vi "MAIN - Template Application.vi"() -> ()   [LabVIEW 2015, in "TLB` Template.lvlib"]
doc: "TLB Prime - Application Template 1.3.0.24\nNorm Kirchner, NI Systems Engineering - NI\nCopyright (c) 2014, NI"
uses:
  TLB` Template.lvlib
  State Declaration.ctl
  System Trigger.ctl
  System Trigger Element.ctl
  <vilib>/Utility/error.llb/DialogTypeEnum.ctl
  Read Termination Message.vi
  Update Message Routing Info.vi
  Create Multiple Messages.vi
  Create Single Message.vi
  TypeDef - SHIFTER.ctl
  Globals.vi
  Send Message.vi
  TLB`_Dependencies.lvlib
  AMC.lvlib
panel:
  out "error out":errorcluster
  # "TLB` Template"
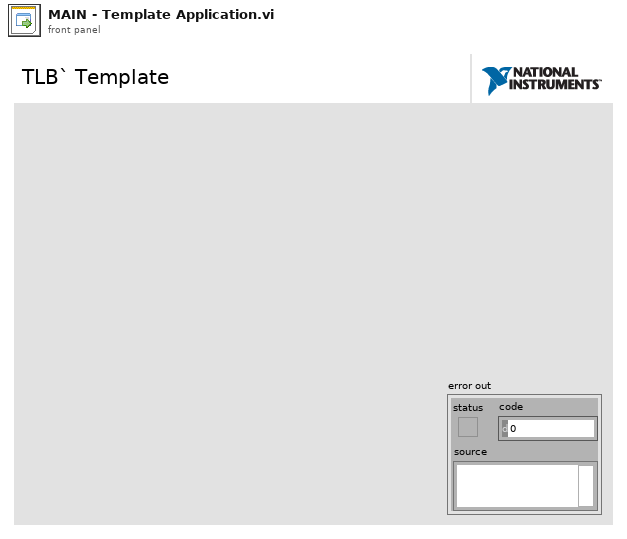
[diagram p1: front panel]
types:
  T1 = typedef "TLB` Template.lvlib/System Trigger.ctl" = enum16{"<None>", "Cache User Parameters", "Close Application"}
  T2 = typedef "TLB` Template.lvlib/State Declaration.ctl" = enum16{"<Startup>", "Idle", "<Shutdown>"}
  T3 = enum16{"Clear SR", "Set Display", "Set Shifter", "Initialize Events", "Init Q"}
  T4 = typedef "TLB` Template.lvlib/TypeDef - SHIFTER.ctl" = cluster{"State":T2, "User Data":cluster{"Active Item Tag":string}, "Display Data":cluster{"Active Item Tag":string}, "User Parameter Controls":refnum<vi>[], "Framework Data":cluster{"Exit Event":T5, "Terminate Error":errorcluster}, "Private Data":cluster{"Active Item Tag":string}}
  T5 = typedef "TLB` Template.lvlib/TLB`_Dependencies.lvlib/Exit Event Ref.ctl" = refnum<user-event>
  T6 = typedef "TLB` Template.lvlib/System Trigger Element.ctl" = cluster{"System Triggers":T1, "Trigger Data":variant}
  T7 = typedef "TLB` Template.lvlib/AMC.lvlib/Message Queue.ctl" = refnum<queue>
  T8 = typedef "DialogTypeEnum.ctl" = enum16{"no dialog", "OK message", "continue or stop message", "auto error handling dialog", "OK message + warnings", "continue/stop + warnings"}
  T9 = enum32{"Invalid", "Standard", "Closed", "Hidden", "Minimized", "Maximized"}
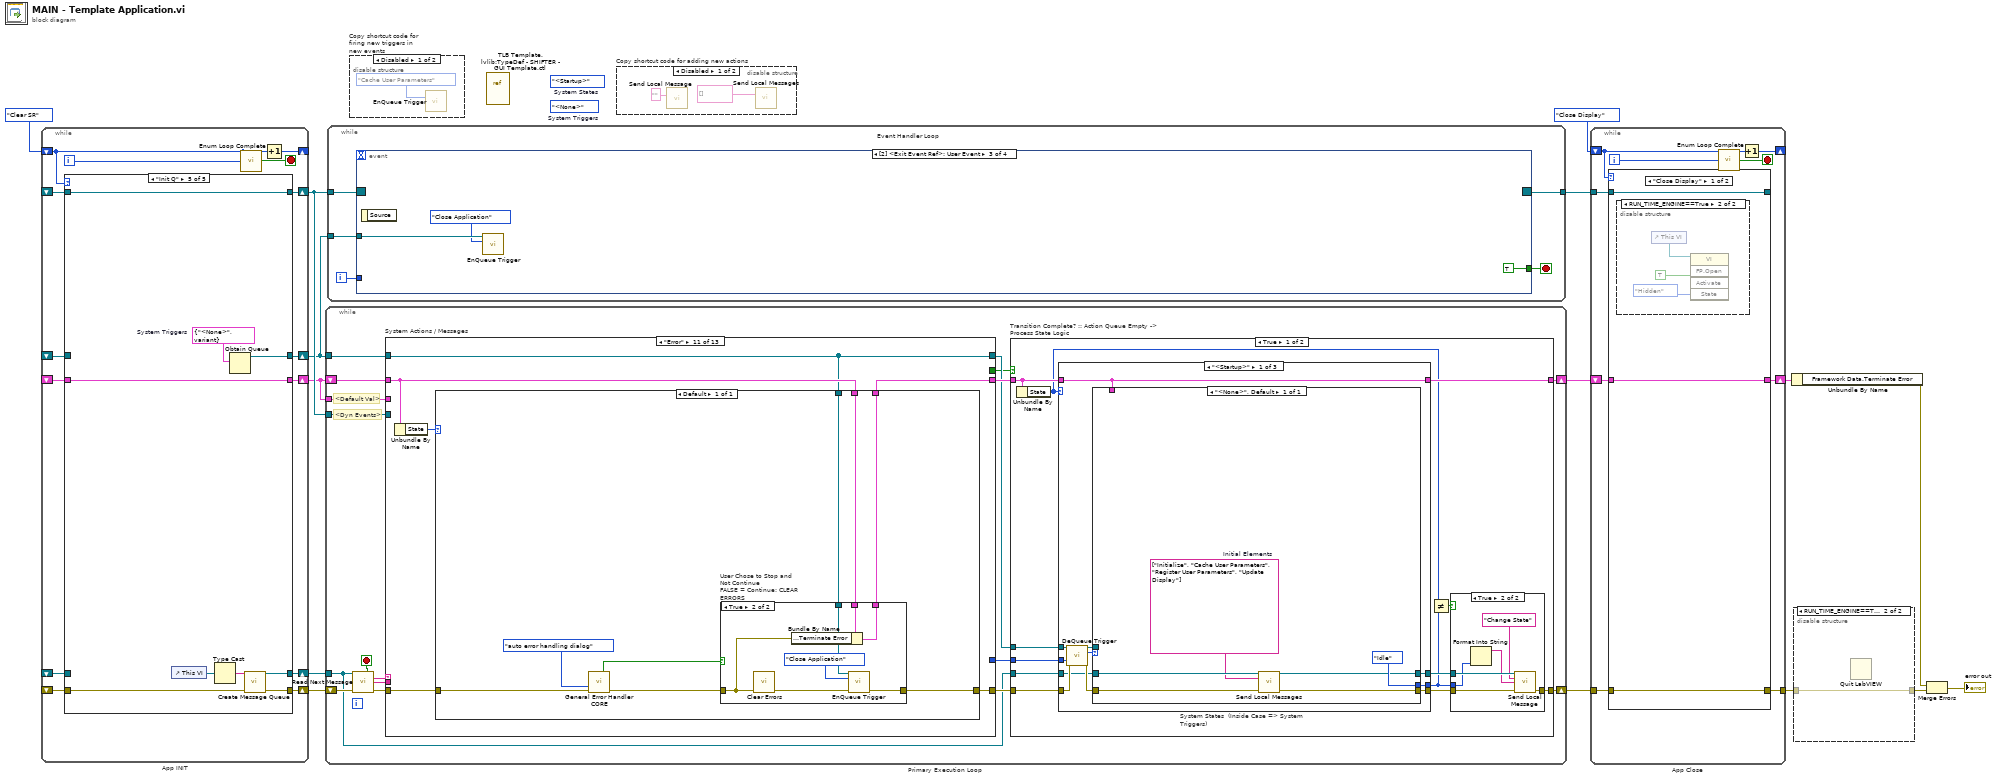
[diagram p0: block diagram]
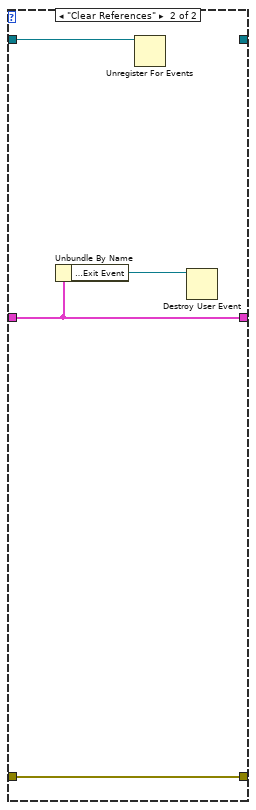
[diagram p6: hidden frame]
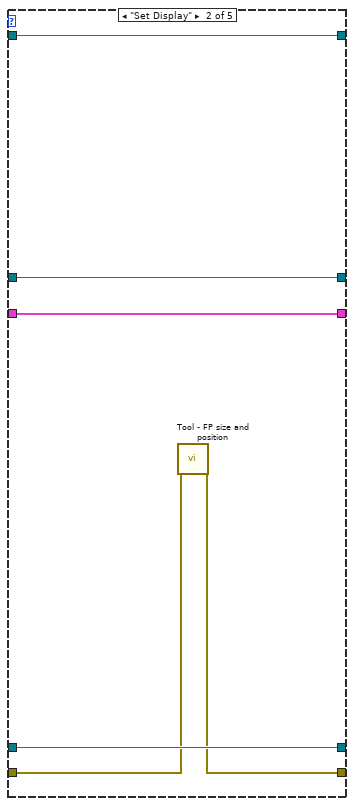
[diagram p8: hidden frame]
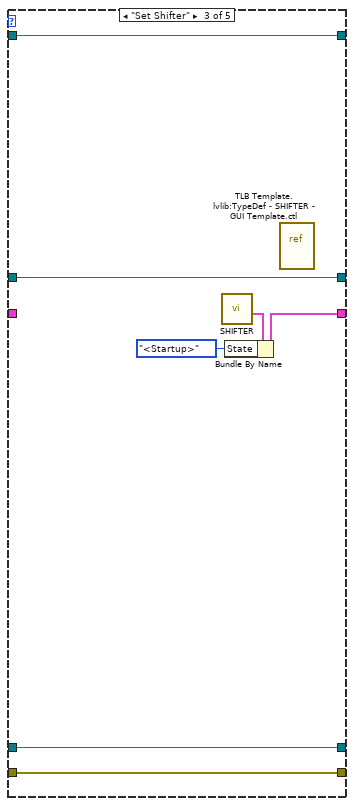
[diagram p9: hidden frame]
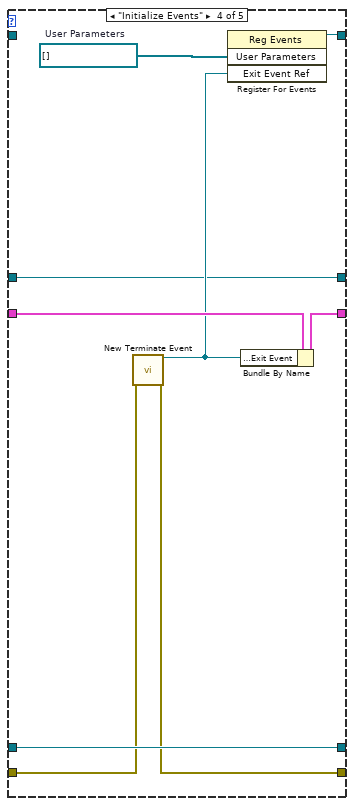
[diagram p10: hidden frame]
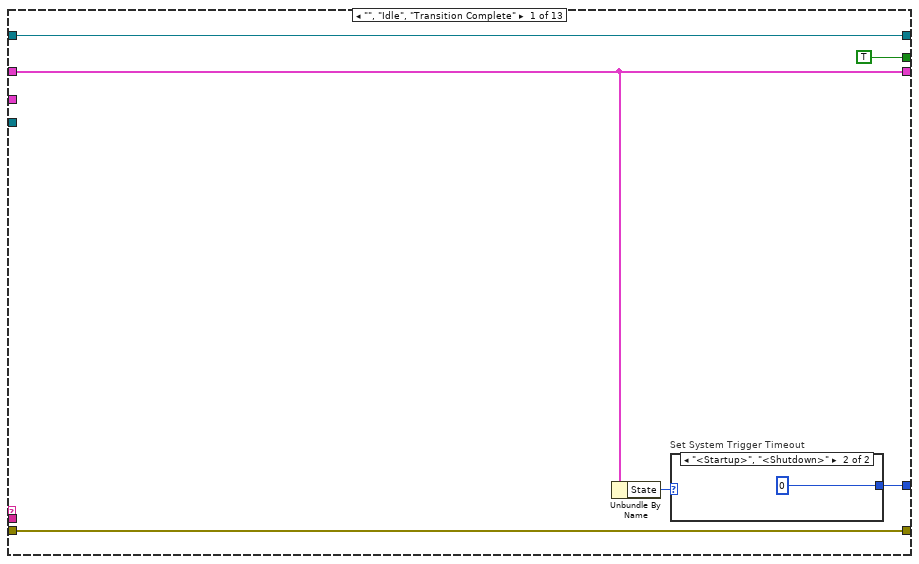
[diagram p11: hidden frame]
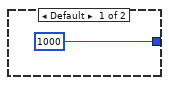
[diagram p12: hidden frame]
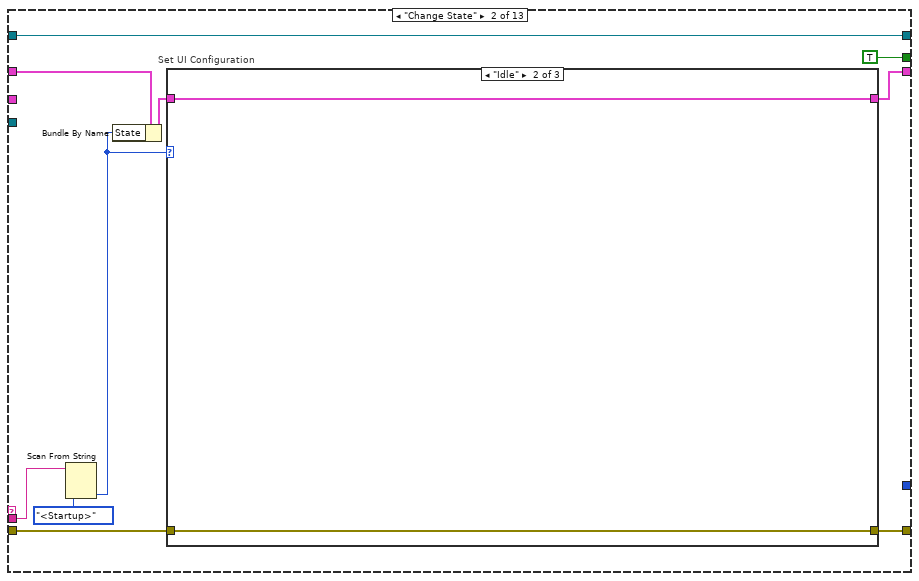
[diagram p13: hidden frame]
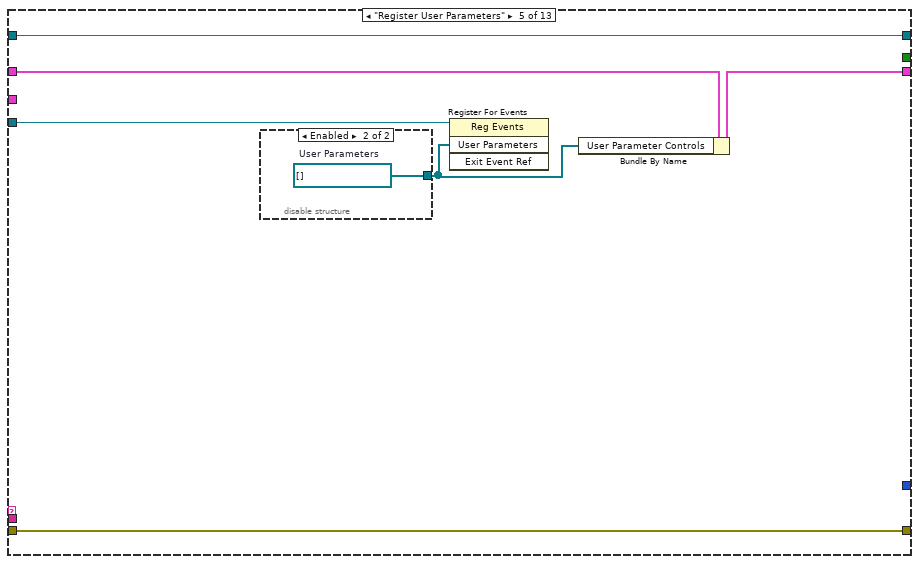
[diagram p18: hidden frame]
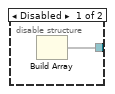
[diagram p19: hidden frame]
diagram:
  (unwired) System_Trigger."<None>"  # System Triggers
  (unwired) State_Declaration."<Startup>"  # System States
  n1 = while "App INIT" {
    shift-right: [w23] -> _
    shift-left: T3."Clear SR" -> [w18]
    shift-right: [w29] -> w9
    shift-left: _ -> [w22]
    shift-right: [w26] -> w8
    shift-left: _ -> [w21]
    shift-right: [w28] -> w11
    shift-left: _ -> [w20]
    shift-right: [w27] -> w1
    shift-left: _ -> [w19]
    shift-right: [w17] -> w2
    shift-left: _ -> [w16]
    i -> [w24]
    stop <- w25 stop-if-true
    n2 = case shown="\"Init Q\"" w18 {
      tunnel: [_ w33 w42 w51 w56] -> w29
      tunnel: [_ w31 w41 w44 w55] -> w26
      tunnel: [_ w35 w36 w48 w54] -> w27
      tunnel: [_ w34 w40 w47 w60] -> w28
      tunnel: w22 -> [_ w33 w42 w51 _]
      tunnel: w21 -> [_ w32 w41 w45 w59]
      tunnel: w20 -> [_ w34 w40 _ w60]
      tunnel: w19 -> [_ w35 _ w49 w54]
      tunnel: [_ w30 w39 w43 w58] -> w17
      tunnel: w16 -> [_ w30 w39 w43 _]
      frame "Clear SR" {
      }
      frame "Set Display" {
        n3 = call "Tool - FP size and position.vi"("error in (no error)"=w32) -> ("error out"=w31:errorcluster)  [unwired: 7 in, 11 out]
      }
      frame "Set Shifter" {
        n4 = call "SHIFTER.vi"() -> ("SHIFTER DATA"=w37:T4)  [unwired: 15 in]
        n5 = Bundle By Name(cluster=w37, "State"=State_Declaration."<Startup>") -> (w36:T4)
        n6 = vi-ref "TLB Template.lvlib:TypeDef - SHIFTER - GUI Template.ctl"() -> ()  [unwired: 1 out]
      }
      frame "Initialize Events" {
        w50 = refnum<vi>[] []  # User Parameters
        n7 = call "New Terminate Event.vi"("error in (no error)"=w45) -> ("Exit Event Ref"=w46:T5, "error out"=w44:errorcluster)  [unwired: 13 in]
        n8 = register-events(w50, w46) -> (reference out=w47:refnum<event-registration>)  [unwired: 2 in, 1 out]
        n9 = Bundle By Name(cluster=w49, "Framework Data.Exit Event"=w46) -> (w48:T4)
      }
      frame "Init Q" {
        w57 = T6 {"System Triggers"=enum."<None>", "Trigger Data"=variant}  # System Triggers
        n10 = control-ref of="This VI"() -> (w53:refnum<vi>)
        n11 = Type Cast(x=w53) -> (*(type *) &x=w52:string)  [unwired: 1 in]
        n12 = Obtain Queue(element data type=w57) -> (queue out=w58:refnum<queue>)  [unwired: 4 in, 2 out]
        n13 = call "Create Message Queue.vi"("message queue name"=w52, "error in"=w59) -> ("message queue out"=w56:T7, "error out"=w55:errorcluster)  [unwired: 12 in]
      }
    }
    n14 = call "Enum Loop Complete.vi"("Current State Enum"=w18, "Itteration"=w24) -> ("Loop Complete?"=w25:bool)  [unwired: 13 out]
    n15 = Increment(x=w18) -> (x+1=w23:T3)
  }
  n16 = while "Primary Execution Loop" {
    shift-right: [w67] -> w15
    shift-left: w8 -> [w74]
    shift-right: [w70] -> w14
    shift-left: w1 -> [w77]
    tunnel: w1 -> [w76]
    tunnel: w9 -> [w65]
    tunnel: w11 -> [w75]
    tunnel: w2 -> [w66]
    stop <- w72 stop-if-true
    # "<Dyn Events>"
    # "<Default Val>"
    n17 = call "Read Next Message.vi"("message queue in"=w65, "error in"=w74) -> ("exit process?"=w72:bool, "message name"=w71:string, "message value"=w62:string, "error out"=w73:errorcluster)  [unwired: 6 in, 4 out]
    n18 = case "System Actions / Messages" shown="\"Error\"" w71 {
      selector: w71 -> [_ _ _ _ _ _ _ _ _ _ _ _ w166]
      tunnel: [w83 w90 w104 w105 w113 w118 w121 w126 w129 w132 w137 w160 w170] -> w68
      tunnel: w73 -> [w83 w89 w104 w105 w113 w118 w121 w126 w129 w132 w138 w159 w171]
      tunnel: w77 -> [w78 w86 w103 w107 w112 w117 w123 w125 w128 w131 w135 w163 w172]
      tunnel: w76 -> [_ _ _ _ _ _ _ _ _ _ _ _ _]
      tunnel: [w78 w88 w103 w107 w111 w117 w122 w125 w128 w131 w136 w163 w172] -> w69
      tunnel: [w79 _ _ _ _ _ _ _ _ _ _ _ _] -> w61
      tunnel: w75 -> [_ _ _ _ w110 _ _ _ _ _ _ _ _]
      tunnel: [w81 w94 w102 w106 w109 w116 w120 w124 w127 w130 w133 w157 w164] -> w64
      tunnel: w66 -> [w81 w94 w102 w106 w109 w116 w120 w124 w127 w130 w133 w157 w164]
      tunnel: [TRUE TRUE _ _ _ _ _ _ _ _ _ _ _] -> w63
      tunnel: w62 -> [_ w93 _ _ _ _ _ _ _ _ _ _ _]
      frame "", "Idle", "Transition Complete" {
        n19 = Unbundle By Name(w78) -> ("State"=w80:T2)
        n20 = case "Set System Trigger Timeout" shown="\"<Startup>\", \"<Shutdown>\"" w80 {
          tunnel: [1000 0] -> w79
          frame Default {
          }
          frame "<Startup>", "<Shutdown>" {
          }
        }
      }
      frame "Change State" {
        n21 = Scan From String(input string=w93, default 1=State_Declaration."<Startup>" ("State")) -> (output 1=w91:T2)  [unwired: 3 in, 3 out]
        n22 = Bundle By Name(cluster=w86, "State"=w91) -> (w87:T4)
        n23 = case "Set UI Configuration" shown="\"Idle\"" w91 {
          tunnel: [w96 w99 w101] -> w90
          tunnel: w89 -> [w96 w99 w101]
          tunnel: [w97 w98 w100] -> w88
          tunnel: w87 -> [w97 w98 w100]
          frame "<Startup>" {
          }
          frame "Idle" {
          }
          frame "<Shutdown>" {
          }
        }
      }
      frame "/*********Initialize********/" {
      }
      frame "Initialize" {
      }
      frame "Register User Parameters" {
        n24 = disable-structure shown="Enabled" {
          disable-tunnel: [w114 w115] -> w108
          frame Disabled {
            n25 = Build Array() -> (w114:void[])  [unwired: 3 in]
          }
          frame Enabled {
            w115 = refnum<vi>[] []  # User Parameters
          }
        }
        n26 = register-events(reference=w110, w108) -> ()  [unwired: 2 in, 2 out]
        n27 = Bundle By Name(cluster=w112, "User Parameter Controls"=w108) -> (w111:T4)
      }
      frame "/*********Display Updates********/" {
      }
      frame "Cache User Parameters" {
        n28 = Bundle By Name(cluster=w123, "User Data.Active Item Tag"="") -> (w122:T4)
      }
      frame "Update Display" {
      }
      frame "/*********Primary Execution********/" {
      }
      frame "/*********Shutdown********/" {
      }
      frame "Error" {
        n29 = Unbundle By Name(w135) -> ("State"=w134:T2)
        n30 = case shown="Default" w134 {
          tunnel: w138 -> [w146]
          tunnel: [w145] -> w137
          tunnel: w135 -> [w142]
          tunnel: [w141] -> w136
          tunnel: w133 -> [w139]
          frame Default {
            n31 = call <vilib>:"General Error Handler CORE.vi"("type of dialog (OK msg:1)"=DialogTypeEnum."auto error handling dialog", "error in (no error)"=w146) -> ("stop event propagated"=w144:bool, "error out"=w140:errorcluster)  [unwired: 12 out]
            n32 = case "User Chose to Stop and Not Continue\nFALSE = Continue: CLEAR ERRORS" shown="True" w144 {
              tunnel: [w147 w152] -> w145
              tunnel: w140 -> [w148 w154]
              tunnel: w142 -> [w149 w156]
              tunnel: [w149 w155] -> w141
              tunnel: w139 -> [_ w153]
              frame False {
                n33 = call <vilib>:"Clear Errors.vi"("error in (no error)"=w148) -> ("error out"=w147:errorcluster)  [unwired: 1 in, 5 out]
              }
              frame True {
                n34 = call <vilib>:"Clear Errors.vi"("error in (no error)"=w154) -> ("error out"=w151:errorcluster)  [unwired: 1 in, 5 out]
                n35 = Bundle By Name(cluster=w156, "Framework Data.Terminate Error"=w154) -> (w155:T4)
                n36 = call "EnQueue Trigger.vi"("Queue in"=w153, "System Triggers"=System_Trigger."Close Application", "error in (no error)"=w151) -> ("error out"=w152:errorcluster)  [unwired: 11 in, 1 out]
              }
            }
          }
        }
      }
      frame "Exit" {
        w158 = refnum<class> refnum  # event data
        # "Don't wire 'Error In'\nMust Execute Regardless"
        n37 = Unbundle By Name(w163) -> ("Framework Data.Exit Event"=w162:T5)  [unwired: 1 out]
        n38 = Generate User Event(user event=w162, event data cluster=w158) -> (error out=w161:errorcluster)  [unwired: 2 in, 1 out]
        n39 = Merge Errors(w161, w159) -> (w160:errorcluster)
      }
      frame Default {
        w168 = 1 items=["No error", "Argument error", "Memory is full", "Out of zone", "End of file", "File already open", "Generic file I/O error", "File not found", "File permission error", "Disk is full", "Duplicate path", "Too many files open", "System feature not enabled", "Resource file not found", "Cannot add resource", "Resource not found", "Image not found", "Image memory error", "Pen does not exist", "Config type invalid", "Config token not found", "Config parse error", "Config memory error", "Bad external code format", "Bad external code offset", "External code not present", "Null window", "Destroy window error", "Null menu", "Print aborted", "Bad print record", "Print driver error", "Windows error during printing", "Memory error during printing", "Print dialog error", "Generic print error", "Invalid device refnum", "Device not found", "Device parameter error", "Device unit error", "Cannot open device", "Device call aborted", "Generic error", "Cancelled by user", "Object ID too low", "Object ID too high", "Object not in heap", "Unknown heap", "Unknown object (invalid DefProc)", "Unknown object (DefProc not in table)", "Message out of range", "Invalid (null) method", "Unknown message", "Manager call not supported", "Bad address", "Network operation in progress", "Network operation timed out", "Connection is busy", "Network attribute not supported", "Network error", "Address in use", "System out of memory", "Connection aborted", "Connection refused", "Not connected", "Already connected", "Connection closed", "Initialization error (interapplication manager)", "Bad occurrence", "Wait on unbound occurrence handler", "Occurrence queue overflow", "Datalog type conflict", "Unused", "Unrecognized type (interapplication manager)", "Memory corrupt", "Failed to make temporary DLL", "Old CIN version", "Drag socket not found", "Failed to load drop-object", "Failed to register OLE object", "Failed to release OLE object", "Format specifier type mismatch", "Unknown format specifier", "Too few format specifiers", "Too many format specifiers", "Scan failed", "Newer CIN version", "Error converting to variant", "Runtime menu error", "Password tampered", "Variant attribute not found", "Incompatible variant data type", "Event data is not available", "Event Store is not present", "Occurrence is not found", "Event Queue is not created", "Event info is not available", "Refnum passed is NULL", "Error retrieving Class GUID", "Error retrieving CoClass GUID", "Error retrieving TypeLib GUID.", "Bad built application magic bytes.", "Specific driver is different from the specific driver associated with the Logical Name.", "There is no session opened to the class driver.", "Max Error", "MAX - Error with config objects", "MAX - Error loading configuration", "MAX - Group not supported"]
        w169 = TRUE  # status
        n40 = Format Into String(format string="DEVELOPER ERROR:\nImproper Action Requested\n================\nAction {%s} does not exist within this architecture\n\nCheck for spelling and case errors" ("source"), w166) -> (resulting string=w167:string)  [unwired: 2 in, 1 out]
        n41 = Bundle By Name(cluster=w171, "status"=w169, "code"=w168, "source"=w167) -> (w170:errorcluster)
      }
    }
    n42 = case "Transition Complete? :: Action Queue Empty -> Process State Logic" shown="True" w63 {
      tunnel: [w184 w254] -> w70
      tunnel: w69 -> [w174 w254]
      tunnel: w68 -> [w183 w253]
      tunnel: w65 -> [w182 _]
      tunnel: [w178 w253] -> w67
      tunnel: w64 -> [w181 _]
      tunnel: w61 -> [w175 _]
      frame True {
        n43 = Unbundle By Name(w174) -> ("State"=w173:T2)
        n44 = case "System States  (Inside Case => System Triggers)" shown="\"<Startup>\"" w173 {
          selector: w173 -> [_ w213 _]
          tunnel: [w200 w219 w244] -> w184
          tunnel: w174 -> [w200 w219 w244]
          tunnel: w183 -> [w194 w211 w238]
          tunnel: w182 -> [w192 w215 w236]
          tunnel: [w199 w218 w243] -> w179
          tunnel: w181 -> [w202 w220 w246]
          tunnel: [w198 w217 w242] -> w180
          tunnel: [w197 w216 w241] -> w177
          tunnel: w175 -> [w196 w209 w240]
          frame "<Startup>" {
            n45 = call "DeQueue Trigger.vi"("Queue in"=w202, "Timeout (0)"=w196, "error in (no error)"=w194) -> ("Queue out"=w195:refnum<queue>, "System Triggers"=w201:T1, "error out"=w193:errorcluster)  [unwired: 9 in, 1 out]
            n46 = case shown="\"<None>\", Default" w201 {
              tunnel: w200 -> [_]
              tunnel: [w206] -> w199
              tunnel: w193 -> [w207]
              tunnel: w192 -> [w205]
              tunnel: [w204] -> w198
              tunnel: [State_Declaration."Idle" ("State")] -> w197
              tunnel: w195 -> [_]
              frame "<None>", Default {
                w203 = string[] ["Initialize", "Cache User Parameters", "Register User Parameters", "Update Display"]  # Initial Elements
                n47 = call "Send Local Messages.vi"("message queue in"=w205, "message names"=w203, "error in"=w207) -> ("message queue out"=w204:T7, "error out"=w206:errorcluster)  [unwired: 10 in, 1 out]
              }
            }
          }
          frame "Idle" {
            n48 = call "DeQueue Trigger.vi"("Queue in"=w220, "Timeout (0)"=w209, "error in (no error)"=w211) -> ("Queue out"=w214:refnum<queue>, "System Triggers"=w212:T1, "error out"=w210:errorcluster)  [unwired: 9 in, 1 out]
            n49 = case shown="\"Cache User Parameters\"" w212 {
              tunnel: w219 -> [_ _ _ _]
              tunnel: [w221 w225 w229 w234] -> w218
              tunnel: w210 -> [w221 w225 w232 w234]
              tunnel: w215 -> [w222 w226 w231 w235]
              tunnel: [w222 w226 w230 w235] -> w217
              tunnel: [State_Declaration."Idle" ("State") State_Declaration."<Shutdown>" ("State") w227 State_Declaration."Idle" ("State")] -> w216
              tunnel: w214 -> [_ _ _ _]
              tunnel: w213 -> [_ _ w227 _]
              frame "<None>" {
              }
              frame "Close Application" {
              }
              frame "Cache User Parameters" {
                n50 = call "Send Local Message.vi"("message queue in"=w231, "message name"="Cache User Parameters" ("Message Name"), "error in"=w232) -> ("message queue out"=w230:T7, "error out"=w229:errorcluster)  [unwired: 10 in, 1 out]
              }
              frame Default {
              }
            }
          }
          frame "<Shutdown>" {
            n51 = call "DeQueue Trigger.vi"("Queue in"=w246, "Timeout (0)"=w240, "error in (no error)"=w238) -> ("Queue out"=w239:refnum<queue>, "System Triggers"=w245:T1, "error out"=w237:errorcluster)  [unwired: 9 in, 1 out]
            n52 = case shown="\"<None>\", Default" w245 {
              tunnel: w244 -> [_]
              tunnel: [w247] -> w243
              tunnel: w237 -> [w249]
              tunnel: w236 -> [w250]
              tunnel: [w248] -> w242
              tunnel: [State_Declaration."<Shutdown>" ("State")] -> w241
              tunnel: w239 -> [_]
              frame "<None>", Default {
                n53 = call "Send Local Messages.vi"("message queue in"=w250, "message names"=string[] ["Exit"], "error in"=w249) -> ("message queue out"=w248:T7, "error out"=w247:errorcluster)  [unwired: 10 in, 1 out]
              }
            }
          }
        }
        n54 = Not Equal?(x=w173, y=w177) -> (x != y?=w176:bool)
        n55 = case shown="True" w176 {
          tunnel: w180 -> [_ w191]
          tunnel: w179 -> [w185 w190]
          tunnel: [w185 w189] -> w178
          tunnel: w177 -> [_ w187]
          frame False {
          }
          frame True {
            n56 = Format Into String(w187) -> (resulting string=w186:string)  [unwired: 3 in, 1 out]
            n57 = call "Send Local Message.vi"("message queue in"=w191, "message name"="Change State" ("Message Name"), "message value"=w186, "error in"=w190) -> ("error out"=w189:errorcluster)  [unwired: 9 in, 2 out]
          }
        }
      }
      frame False {
      }
    }
  }
  n58 = while "Event Handler Loop" {
    tunnel: w11 -> [w258]
    tunnel: [w257] -> w13
    tunnel: w2 -> [w255]
    i -> [w256]
    stop <- w259 stop-if-true
    n59 = event shown="[2] <Exit Event Ref>: User Event" {
      selector: w258 -> [_ _ _ _]
      dyn-events: [_ _ _ _] -> w257
      timeout: _ -> [_ _ _ _]
      tunnel: [_ _ TRUE ("NewVal") _] -> w259
      tunnel: w256 -> [_ _ _ _]
      tunnel: w255 -> [w261 _ w273 w277]
      event Panel Close? {
        w262 = TRUE  # Discard?
        n60 = event-data() -> ()  [unwired: 2 out]
        n61 = call "EnQueue Trigger.vi"("Queue in"=w261, "System Triggers"=System_Trigger."Close Application") -> ()  [unwired: 12 in, 2 out]
        n62 = event-data("Discard?"=w262) -> ()  [unwired: 1 in, 1 out]
      }
      event Mouse Down {
        n63 = event-data() -> ("Button"=w267:u16, "Mods"=w268:cluster{"Double Click":bool, "Menu Key":bool})  [unwired: 1 out]
        n64 = Unbundle By Name(w268) -> ("Double Click"=w264:bool)
        n65 = Equal?(x=u16 2, y=w267) -> (x = y?=w265:bool)
        n66 = And(x=w265, y=w264) -> (x .and. y?=w263:bool)
        n67 = case "Toggle Menu Visibility :: double RIGHT click on logo" shown="True" w263 {
          frame False {
          }
          frame True {
            n68 = property class="VI"() -> (reference out=w271:refnum<vi>, "TB.Visible"=w269:bool)  [unwired: 2 in, 1 out]
            n69 = Not(x=w269) -> (.not. x?=w270:bool)
            n70 = property class="VI"(reference=w271, "TB.Visible"=w270) -> ()  [unwired: 1 in, 2 out]
          }
        }
      }
      event User Event {
        n71 = event-data() -> ()  [unwired: 2 out]
        n72 = call "EnQueue Trigger.vi"("Queue in"=w273, "System Triggers"=System_Trigger."Close Application") -> ()  [unwired: 12 in, 2 out]
      }
      event Value Change {
        n73 = event-data() -> ()  [unwired: 2 out]
        n74 = call "EnQueue Trigger.vi"("Queue in"=w277, "System Triggers"=System_Trigger."Cache User Parameters") -> ("Queue out"=w276:refnum<queue>)  [unwired: 12 in, 1 out]
        n75 = event "use this event case to register a SPEICIFIC 'User Parameter' for a SPECIFIC action" shown="[0] Timeout" {
          selector: _ -> [_]
          dyn-events: _ -> [_]
          timeout: 0 -> [_]
          tunnel: w276 -> [_]
          event Timeout {
            n76 = event-data() -> ()  [unwired: 1 in, 1 out]
          }
        }
      }
    }
  }
  n77 = disable-structure "Copy shortcut code for firing new triggers in new events" shown="Disabled" {
    frame Disabled {
      n78 = call "EnQueue Trigger.vi"("System Triggers"=System_Trigger."Cache User Parameters") -> ()  [unwired: 13 in, 2 out]
    }
    frame Enabled {
    }
  }
  n79 = vi-ref "TLB Template.lvlib:TypeDef - SHIFTER - GUI Template.ctl"() -> ()  [unwired: 1 out]
  n80 = disable-structure "Copy shortcut code for adding new actions" shown="Disabled" {
    frame Disabled {
      n81 = call "Send Local Message.vi"("message name"="") -> ()  [unwired: 12 in, 3 out]
      n82 = call "Send Local Messages.vi"("message names"=string[] []) -> ()  [unwired: 12 in, 3 out]
    }
    frame Enabled {
    }
  }
  n83 = while "App Close" {
    shift-right: [w288] -> _
    shift-left: enum16{"Close Display", "Clear References"}."Close Display" -> [w287]
    tunnel: w13 -> [w285]
    tunnel: w15 -> [w286]
    tunnel: [w283] -> w7
    shift-right: [w282] -> w5
    shift-left: w14 -> [w284]
    i -> [w289]
    stop <- w290 stop-if-true
    n84 = case shown="\"Close Display\"" w287 {
      tunnel: [w292 w300] -> w283
      tunnel: [w291 w299] -> w282
      tunnel: [w293 _] -> _
      tunnel: w286 -> [w292 w300]
      tunnel: w285 -> [w293 w297]
      tunnel: w284 -> [w291 w299]
      frame "Close Display" {
        n85 = disable-structure shown="RUN_TIME_ENGINE==True" {
          frame condition #0 (active) {
          }
          frame condition #1 {
            n86 = control-ref of="This VI"() -> (w294:refnum<vi>)
            n87 = invoke class="VI" method="FP.Open"(reference=w294, "Activate"=TRUE ("Activate?"), "State"=T9."Hidden") -> ()  [unwired: 2 in, 5 out]
          }
        }
      }
      frame "Clear References" {
        n88 = Unbundle By Name(w299) -> ("Framework Data.Exit Event"=w298:T5)
        n89 = Unregister For Events(event registration refnum=w297) -> ()  [unwired: 1 in, 1 out]
        n90 = Destroy User Event(user event=w298) -> ()  [unwired: 1 in, 1 out]
      }
    }
    n91 = call "Enum Loop Complete.vi"("Current State Enum"=w287, "Itteration"=w289) -> ("Loop Complete?"=w290:bool)  [unwired: 13 out]
    n92 = Increment(x=w287) -> (x+1=w288:enum16{"Close Display", "Clear References"})
  }
  n93 = Unbundle By Name(w5) -> ("Framework Data.Terminate Error"=w3:errorcluster)
  n94 = disable-structure shown="RUN_TIME_ENGINE==True" {
    disable-tunnel: [w301 w302] -> w4
    disable-tunnel: w7 -> [w301 w302]
    frame condition #0 (active) {
    }
    frame condition #1 {
      n95 = Quit LabVIEW() -> ()  [unwired: 1 in]
    }
  }
  n96 = Merge Errors(w3, w4) -> (→"error out":errorcluster)
